vi "PlaneFit.vi"(7 "Reset Clicks":bool, 8 "Y PEN":dbl, 9 "Z":dbl, 10 "Nano Z":dbl, 11 "X":dbl) -> (2 "Plane Height (m)":dbl, 3 "Clicks":dbl)   [LabVIEW 2017]
uses:
  <userlib>/HapticSTM/Feedbackless - Testdata/Project/feedbackless.lvproj/HapticSTM.lvlib
  <userlib>/HapticSTM/Feedbackless - Testdata/Project/feedbackless.lvproj/GlobalClicksHeight.vi
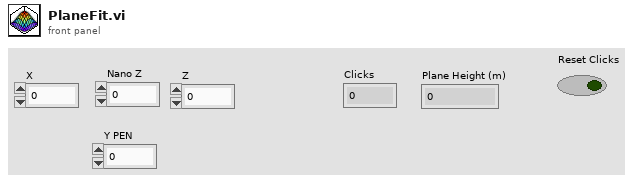
[diagram p1: front panel]
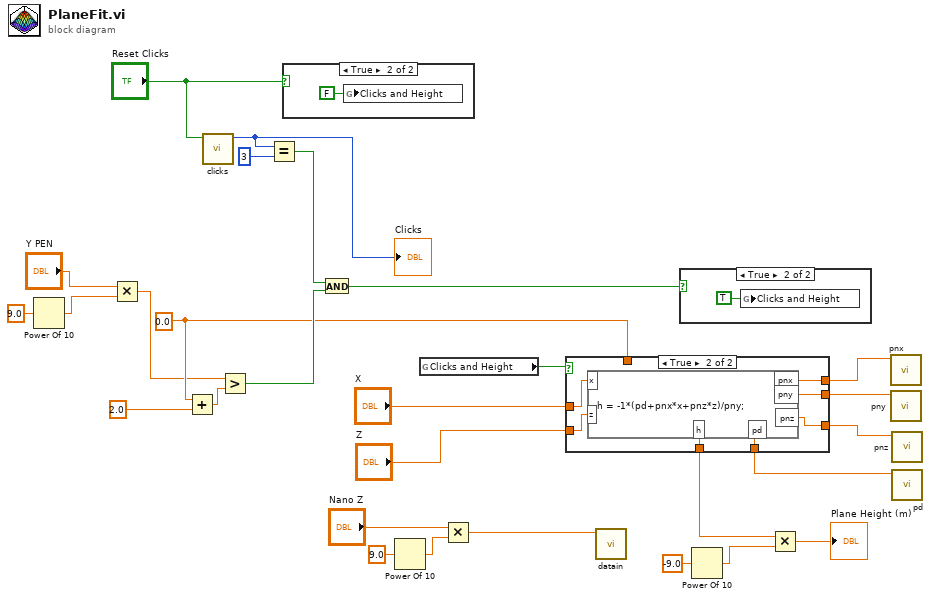
[diagram p0: block diagram]
diagram:
  w15 = 0.0 ("Plane Height")
  n1 = Power Of 10(x=9.0) -> (10^x=w12:dbl)
  n2 = Multiply(x="Y PEN", y=w12) -> (x*y=w9:dbl)
  n3 = Add(x=w15, y=2.0) -> (x+y=w17:dbl)
  n4 = call <userlib>:"clicks.vi"("reset"="Reset Clicks") -> ("function return"=w26:i32)  [unwired: 10 in]
  "Clicks" <- w26
  n5 = Greater?(x=w9, y=w17) -> (0:w18:bool)
  n6 = Equal?(x=w26, y=3) -> (x = y?=w19:bool)
  n7 = case shown="True" "Reset Clicks" {
    frame False {
    }
    frame True {
      n8 = global write "GlobalClicksHeight.vi" "Clicks and Height"(FALSE ("Clicks and Height")) -> ()
    }
  }
  n9 = And(x=w19, y=w18) -> (x .and. y?=w14:bool)
  n10 = Power Of 10(x=9.0) -> (10^x=w8:dbl)
  n11 = global read "GlobalClicksHeight.vi" "Clicks and Height"() -> (w13:bool)
  n12 = Multiply(x="Nano Z", y=w8) -> (x*y=w3:dbl)
  n13 = call <userlib>:"datain.vi"("output"=w3) -> ()  [unwired: 11 in]
  n14 = case shown="True" w14 {
    frame False {
    }
    frame True {
      n15 = global write "GlobalClicksHeight.vi" "Clicks and Height"(TRUE ("Clicks and Height")) -> ()
    }
  }
  n16 = Power Of 10(x=-9.0) -> (10^x=w22:dbl)
  n17 = call <userlib>:"pnx.vi"() -> ("function return"=w24:dbl)  [unwired: 11 in]
  n18 = call <userlib>:"pny.vi"() -> ("function return"=w23:dbl)  [unwired: 11 in]
  n19 = call <userlib>:"pnz.vi"() -> ("function return"=w28:dbl)  [unwired: 11 in]
  n20 = call <userlib>:"pd.vi"() -> ("function return"=w27:dbl)  [unwired: 11 in]
  n21 = case shown="True" w13 {
    tunnel: "X" -> [_ w38]
    tunnel: w24 -> [_ w36]
    tunnel: w23 -> [_ w35]
    tunnel: w28 -> [_ w34]
    tunnel: w27 -> [_ w33]
    tunnel: "Z" -> [_ w37]
    tunnel: [w31 w32] -> w4
    tunnel: w15 -> [w31 _]
    frame False {
    }
    frame True {
      n22 = formula code="h = -1*(pd+pnx*x+pnz*z)/pny;"("x"=w38, "z"=w37, "pnx"=w36, "pnz"=w34, "pd"=w33, "pny"=w35) -> ("h"=w32:dbl)
    }
  }
  n23 = Multiply(x=w4, y=w22) -> (x*y=→"Plane Height (m)":dbl)
